vi "Update_states.vi"(8 "error in (no error)":errorcluster, 9 "State-status":string, 11 "ATM_UI_Controller in":refnum<class "ATM_UI_Controller.lvclass">) -> (0 "error out":errorcluster, 3 "ATM_UI_Controller out":refnum<class "ATM_UI_Controller.lvclass">)   [LabVIEW 2025, in "ATM_UI_Controller.lvlib" / "ATM_UI_Controller.lvclass"]
uses:
  ATM_UI_Controller.lvclass
  ATM_UI_Controller.lvclass/ATM_UI_Controller.ctl
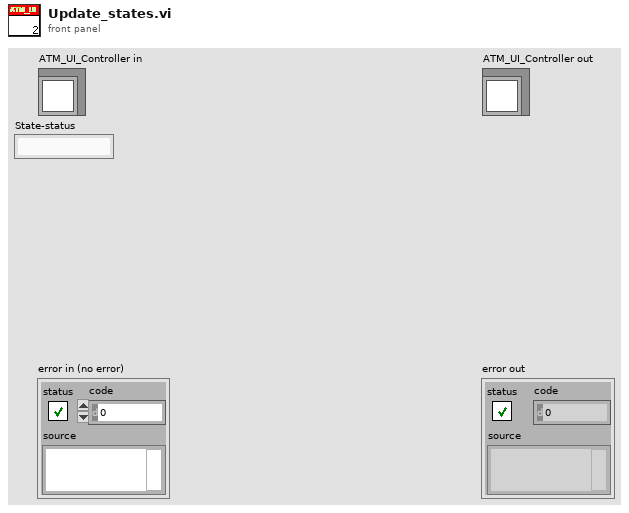
[diagram p1: front panel]
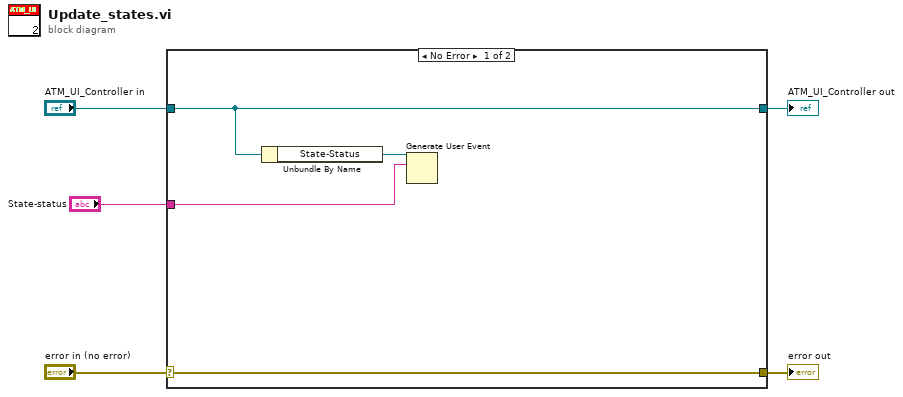
[diagram p0: block diagram]
diagram:
  n1 = case shown="No Error" "error in (no error)" {
    selector: "error in (no error)" -> [w9 w11]
    tunnel: [w9 w11] -> w4
    tunnel: [w8 w10] -> w2
    tunnel: "ATM_UI_Controller in" -> [w8 w10]
    tunnel: "State-status" -> [w6 _]
    frame No Error {
      n2 = Unbundle By Name(w8) -> ("State-Status"=w7:refnum<user-event>)
      n3 = Generate User Event(user event=w7, event data cluster=w6) -> ()  [unwired: 2 in, 2 out]
    }
    frame Error {
    }
  }
  "error out" <- w4
  "ATM_UI_Controller out" <- w2
